vi "Parse XML and Create Clusters.vi"(6 "Settings Cluster Path":path, 8 "error in":errorcluster, 11 "Document Element":refnum<k20>) -> (0 "error out":errorcluster, 3 "Document Element":refnum<k20>)   [LabVIEW 2026, in "Plugin XML Parser.lvlib"]
uses:
  Plugin XML Parser.lvlib
  <vilib>/xml/Close Reference(Node).vi
  <resource>/objmgr/DOMUserDefRef.rc
  <vilib>/xml/NI_XML.lvlib
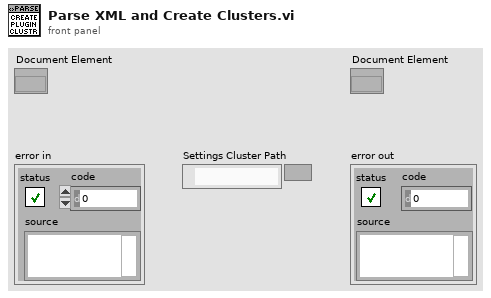
[diagram p1: front panel]
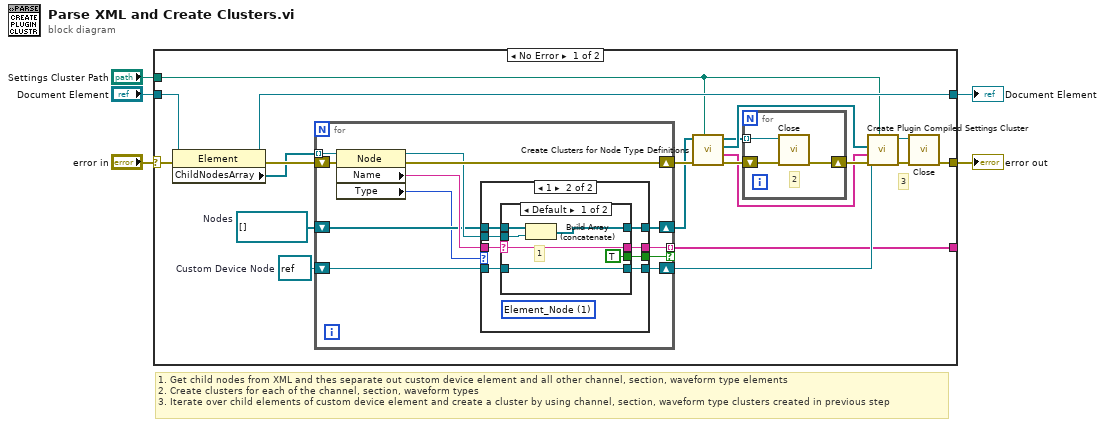
[diagram p0: block diagram]
diagram:
  # "1. Get child nodes from XML and thes separate out custom device element and all other channel, section, waveform type elements\n2. Create clusters for each of the channel, section, waveform types\n3. Iterate over child elements of custom device element and create a cluster by using channel, section, waveform type clusters created in previous step"
  n1 = case shown="No Error" "error in" {
    selector: "error in" -> [w24 w60]
    tunnel: [w21 w60] -> w4
    tunnel: [w18 w59] -> w3
    tunnel: "Document Element" -> [w14 w59]
    tunnel: "Settings Cluster Path" -> [w6 _]
    tunnel: [w7 _] -> _
    frame No Error {
      w15 = refnum<k20> refnum  # Custom Device Node
      w16 = refnum<k20>[] []  # Nodes
      # "3"
      n2 = property class="Element"(reference=w14, error in=w24) -> (reference out=w18:refnum<k20>, error out=w25:errorcluster, "ChildNodesArray"=w17:refnum<k20>[])
      n3 = for {
        tunnel: w17 -> [w38] mode=indexing
        shift-right: [w36] -> w13
        shift-left: w16 -> [w34]
        shift-right: [w33] -> w12
        shift-left: w15 -> [w32]
        shift-right: [w39] -> w23
        shift-left: w25 -> [w40]
        tunnel: [w30] -> w7 mode=indexing if=w29
        n4 = property class="Node"(reference=w38, error in=w40) -> (reference out=w35:refnum<k20>, error out=w39:errorcluster, "Name"=w37:string, "Type"=w31:i32)
        n5 = case shown="1" w31 {
          tunnel: w37 -> [_ w50]
          tunnel: [w42 w49] -> w36
          tunnel: w35 -> [_ w48]
          tunnel: w34 -> [w42 w47]
          tunnel: [w41 w46] -> w33
          tunnel: w32 -> [w41 w45]
          tunnel: [_ w44] -> w30
          tunnel: [_ w43] -> w29
          frame 0, Default {
          }
          frame 1 {
            (unwired) 1 items=["Element_Node"=1, "Attribute_Node"=2, "Text_Node"=3, "CDATASection_Node"=4, "EntityReference_Node"=5, "Entity_Node"=6, "ProcessingInstruction_Node"=7, "Comment_Node"=8, "Document_Node"=9, "DocumentType_Node"=10, "DocumentFragment_Node"=11, "Notation_Node"=12] ("Node Type")
            n6 = case shown="Default" w50 {
              selector: w50 -> [w52 _]
              tunnel: [w55 w57] -> w49
              tunnel: w48 -> [w56 w58]
              tunnel: w47 -> [w54 w57]
              tunnel: [w53 w58] -> w46
              tunnel: w45 -> [w53 _]
              tunnel: [w52 _] -> w44
              tunnel: [TRUE _] -> w43
              frame Default {
                # "1"
                n7 = Build Array (concatenate)(w54, w56) -> (w55:refnum<k20>[])
              }
              frame "customdevice" {
              }
            }
          }
        }
      }
      n8 = call "Create Clusters for Node Type Definitions.vi"("Settings Cluster Path"=w6, "error in"=w23, "Nodes"=w13) -> ("error out"=w20:errorcluster, "Node Types"=w10:string[], "Node Clusters"=w11:refnum<vi>[], "Nodes"=w8:refnum<k20>[])  [unwired: 5 in]
      n9 = for {
        tunnel: w8 -> [w26] mode=indexing
        shift-right: [w27] -> w19
        shift-left: w20 -> [w28]
        # "2"
        n10 = call-poly <vilib>:"Close.vi"("error in (no error)"=w28, "node"=w26) -> ("error out"=w27:errorcluster)  [unwired: 7 in]
      }
      n11 = call "Create Plugin Compiled Settings Cluster.vi"("Settings Cluster Path"=w6, "error in"=w19, "Node Types"=w10, "Node Clusters"=w11, "Node"=w12) -> ("error out"=w22:errorcluster, "Node"=w9:refnum<k20>)  [unwired: 5 in]
      n12 = call-poly <vilib>:"Close.vi"("error in (no error)"=w22, "node"=w9) -> ("error out"=w21:errorcluster)  [unwired: 7 in]
    }
    frame Error {
    }
  }
  "Document Element" <- w3
  "error out" <- w4
